vi "Test MQTT-3.1.2-12.vi"(8 "error in (no error)":errorcluster) -> (0 "error out":errorcluster)   [LabVIEW 2013]
uses:
  source/Control Packets/CONNECT/ConnectFlags -- cluster.ctl
  source/Control Packets/ControlPacket/QualityOfService -- enum.ctl
  source/Control Packets/ControlPacket/ControlPacket.lvclass
  source/Client/Client.lvclass/Client.ctl
  source/Client/Client.lvclass
  <vilib>/addons/_JKI Toolkits/Caraya/classes/Assert/Assert Equal Value_Variant.vi
  <vilib>/addons/_JKI Toolkits/Caraya/classes/Assert/Assert Equal Value and Type_Variant.vi
  source/Control Packets/PUBLISH/PUBLISH.lvclass
  <vilib>/addons/_JKI Toolkits/Caraya/classes/Test/Test.lvclass
  <vilib>/addons/_JKI Toolkits/Caraya/classes/Assert/Assert.lvclass
  source/Control Packets/CONNECT/CONNECT.lvclass
  source/MQTT_Base/MQTT_Base.lvclass
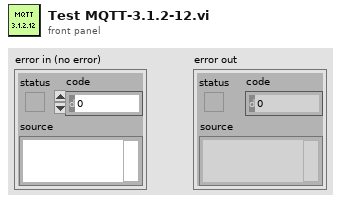
[diagram p1: front panel]
types:
  T1 = typedef "ControlPacket.lvclass/QualityOfService -- enum.ctl" = enum16{"0 (At Most Once)", "1 (At Least Once)", "2 (Exactly Once)"}
  T2 = typedef "CONNECT.lvclass/ConnectFlags -- cluster.ctl" = cluster{"Reserved":bool, "Clean Session":bool, "Will Flag":bool, "Will QoS 1":bool, "Will QoS 2":bool, "Will Retain":bool, "Password Flag":bool, "User Name Flag":bool}
  T3 = cluster{"Will Topic":string, "Will Message":string, "Username":string, "Password":string}
  T4 = typedef "MQTT Server.lvlib/Client.lvclass/Public Events -- cluster.ctl" = cluster{"Connection Status":refnum<user-event>, "Connected":refnum<user-event>, "Application Message":refnum<user-event>}
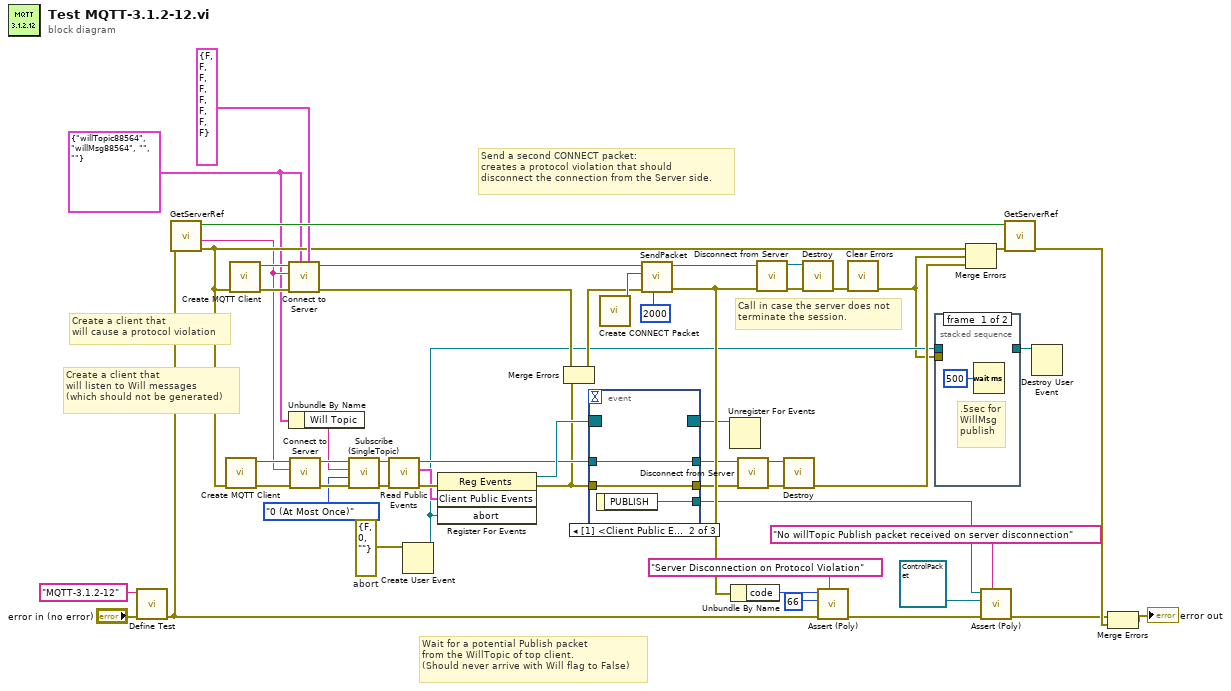
[diagram p0: block diagram]
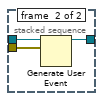
[diagram p2: hidden frame]
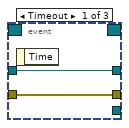
[diagram p3: hidden frame]
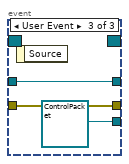
[diagram p4: hidden frame]
diagram:
  w16 = errorcluster {"status"=FALSE, "code"=0, "source"=""}  # abort
  w27 = T3 {"Will Topic"="willTopic88564", "Will Message"="willMsg88564", "Username"="", "Password"=""} ("Payload")
  # "Wait for a potential Publish packet\nfrom the WillTopic of top client.\n(Should never arrive with Will flag to False)"
  # "Create a client that\nwill listen to Will messages\n(which should not be generated)"
  # "Create a client that\nwill cause a protocol violation"
  # "Call in case the server does not\nterminate the session."
  # "Send a second CONNECT packet:\ncreates a protocol violation that should\ndisconnect the connection from the Server side."
  n1 = call <vilib>:"Define Test.vi"("error in (no error)"="error in (no error)", "Label (VI Title)"="MQTT-3.1.2-12") -> ("error out"=w48:errorcluster)  [unwired: 9 in]
  n2 = call "GetServerRef.vi"("error in"=w48) -> ("error out"=w32:errorcluster, "Server address"=w29:string, "Created"=w49:bool)  [unwired: 7 in, 1 out]
  n3 = call "Create MQTT Client.vi"("error in (no error)"=w32) -> ("error out"=w31:errorcluster, "Client out"=w30:refnum<class "Client.lvclass">)  [unwired: 9 in]
  n4 = call "Create MQTT Client.vi"("error in (no error)"=w32) -> ("error out"=w44:errorcluster, "Client out"=w45:refnum<class "Client.lvclass">)  [unwired: 9 in]
  n5 = call "Connect to Server.vi"("Connect Flags"=T2 {"Reserved"=FALSE, "Clean Session"=FALSE, "Will Flag"=FALSE, "Will QoS 1"=FALSE, "Will QoS 2"=FALSE, "Will Retain"=FALSE, "Password Flag"=FALSE, "User Name Flag"=FALSE}, "Payload"=w27, "error in (no error)"=w44, "address (localhost)"=w29, "Client in"=w45) -> ("error out"=w23:errorcluster, "Client out"=w42:refnum<class "Client.lvclass">)  [unwired: 3 in, 2 out]
  n6 = Unbundle By Name(w27) -> ("Will Topic"=w26:string)
  n7 = call "Connect to Server.vi"("error in (no error)"=w31, "address (localhost)"=w29, "Client in"=w30) -> ("error out"=w25:errorcluster, "Client out"=w28:refnum<class "Client.lvclass">)  [unwired: 5 in, 2 out]
  n8 = call "Subscribe (SingleTopic).vi"("error in (no error)"=w25, "QoS"=QualityOfService_--_enum."0 (At Most Once)", "Topic Filter"=w26, "MQTT_Base in"=w28) -> ("error out"=w20:errorcluster, "MQTT_Base out"=w21:refnum<class "Client.lvclass">)  [unwired: 6 in]
  n9 = call "Read Public Events.vi"("error in (no error)"=w20, "Client in"=w21) -> ("error out"=w19:errorcluster, "Client Public Events"=w18:T4, "Client out"=w14:refnum<class "Client.lvclass">)  [unwired: 7 in]
  n10 = Create User Event(user event datatype=w16) -> (user event=w4:refnum<user-event>)  [unwired: 1 in, 1 out]
  n11 = register-events(error in=w19, w18, w4) -> (reference out=w17:refnum<event-registration>, error out=w13:errorcluster)  [unwired: 1 in]
  n12 = Merge Errors(w23, w13) -> (w22:errorcluster)
  n13 = event shown="[1] <Client Public Events.Application Message>: User Event" {
    selector: w17 -> [_ _ _]
    dyn-events: [_ _ _] -> w15
    timeout: _ -> [_ _ _]
    tunnel: [_ w59 refnum<class "ControlPacket.lvclass"> refnum ("ControlPacket.lvclass")] -> w6
    tunnel: w14 -> [w56 w58 w61]
    tunnel: w13 -> [w55 w57 w60]
    tunnel: [w56 w58 w61] -> w10
    tunnel: [w55 w57 w60] -> w9
    event Timeout {
      n14 = event-data() -> ()  [unwired: 1 in, 1 out]
    }
    event User Event {
      n15 = event-data() -> ("PUBLISH"=w59:refnum<class "PUBLISH.lvclass">)  [unwired: 1 in]
    }
    event User Event {
      n16 = event-data() -> ()  [unwired: 1 in, 1 out]
    }
  }
  n17 = call "Create CONNECT Packet.vi"() -> ("CONNECT"=w35:refnum<class "CONNECT.lvclass">)  [unwired: 10 in, 1 out]
  n18 = call "SendPacket.vi"("timeout (0ms : no ack)"=2000, "error in (no error)"=w22, "ControlPacket"=w35, "Client in"=w42) -> ("error out"=w36:errorcluster, "Client out"=w38:refnum<class "Client.lvclass">)  [unwired: 5 in, 1 out]
  n19 = Unregister For Events(event registration refnum=w15) -> ()  [unwired: 1 in, 1 out]
  n20 = Unbundle By Name(w36) -> ("code"=w46:i32)
  n21 = call "Disconnect from Server.vi"("error in (no error)"=w9, "Client in"=w10) -> ("error out"=w12:errorcluster, "Client out"=w11:refnum<class "Client.lvclass">)  [unwired: 7 in, 1 out]
  n22 = call "Disconnect from Server.vi"("error in (no error)"=w36, "Client in"=w38) -> ("error out"=w39:errorcluster, "Client out"=w40:refnum<class "Client.lvclass">)  [unwired: 7 in, 1 out]
  n23 = call-dynamic "Destroy.vi"("error in (no error)"=w12, "Client in"=w11) -> ("error out"=w8:errorcluster)  [unwired: 8 in, 1 out]
  n24 = call-dynamic "Destroy.vi"("error in (no error)"=w39, "Client in"=w40) -> ("error out"=w37:errorcluster)  [unwired: 8 in, 1 out]
  n25 = call-poly <vilib>:"Assert (Poly).vi"("Label"="Server Disconnection on Protocol Violation", "error in (no error)"=w48, "Y"=66 ("code"), "X"=w46) -> ("error out"=w34:errorcluster)  [unwired: 7 in]
  n26 = call <vilib>:"Clear Errors.vi"("error in (no error)"=w37) -> ("error out"=w3:errorcluster)  [unwired: 6 in]
  n27 = stacked-sequence {
    tunnel: w4 -> [_ w66]
    tunnel: w3 -> [_ w65]
    tunnel: [_ w64] -> w2
    frame #0 {
      # ".5sec for\nWillMsg\npublish"
      n28 = Wait (ms)(milliseconds to wait=u32 500) -> ()  [unwired: 1 out]
    }
    frame #1 {
      n29 = Generate User Event(user event=w66, event data cluster=w65) -> (user event out=w64:refnum<user-event>)  [unwired: 2 in, 1 out]
    }
  }
  n30 = Merge Errors(w32, w3, w8) -> (w7:errorcluster)
  n31 = call-poly <vilib>:"Assert (Poly).vi"("Label"="No willTopic Publish packet received on server disconnection", "error in (no error)"=w34, "Y"=refnum<class "ControlPacket.lvclass"> refnum ("ControlPacket.lvclass"), "X"=w6) -> ("error out"=w33:errorcluster)  [unwired: 7 in]
  n32 = call "GetServerRef.vi"("error in"=w7, "Destroy (F)"=w49) -> ("error out"=w47:errorcluster)  [unwired: 6 in, 3 out]
  n33 = Destroy User Event(user event=w2) -> ()  [unwired: 1 in, 1 out]
  n34 = Merge Errors(w33, w47) -> (→"error out":errorcluster)
